vi "Process.vi"(8 "error in":errorcluster, 11 "Sequence Experiment UI":refnum<class "Control Experiment UI.lvclass">) -> (0 "error out":errorcluster, 3 "Sequence Experiment UI out":refnum<class "Control Experiment UI.lvclass">)   [LabVIEW 2019, in "Control Experiment UI.lvclass"]
doc: "---------------------------------------------------------------\nJKI State Machine Objects™\nhttp://jki.net/state-machine-objects/\nCopyright (C) 2005-2015, JKI <info@jki.net>\nALL RIGHTS RESERVEDJKI State Machine Objects (SMO) 1.0.0.5\nJKI - JKI\nCopyright (c) 2016, JKI"
uses:
  Control Experiment UI.lvclass
  <vilib>/JKI/JKI SMO/SMO/SMO.lvclass
  <vilib>/JKI/JKI SMO/SMO/Typedefs/Parent Call--Enum.ctl
  <vilib>/JKI/JKI SMO/SMO.UI/SMO.UI.lvclass
  <userlib>/LevyLab/Instrument Framework/SMOs/Instrument/Instrument.lvclass
  <userlib>/LevyLab/Instrument Framework/SMOs/Instrument UI/Instrument UI.lvclass
  Control Experiment/Control Experiment.lvclass
  <userlib>/LevyLab/Krohn Hite 7008/typedefs/Input Configuration-Enum.ctl
  <userlib>/LevyLab/Krohn Hite 7008/Instrument.KH7008.lvclass
  <userlib>/LevyLab/Instrument Framework/SMOs/Configuration/Configuration.lvclass
  Control Experiment/Private/Control Experiment SM/Typedefs/Instrument--enum.ctl
  Control Experiment/Private/Control Experiment SM/Typedefs/KH Mode-enum.ctl
  <userlib>/LevyLab/Krohn Hite 7008/typedefs/Gain-Enum.ctl
  <userlib>/LevyLab/Krohn Hite 7008/typedefs/Shunt-Enum.ctl
  Typedefs/UI Channels.AO--Cluster.ctl
  Typedefs/UI Channels.KH--Cluster.ctl
  Typedefs/UI Channels.Device--Cluster.ctl
  Typedefs/UI Channels.AI--Cluster.ctl
  Typedefs/UI Channels--Cluster.ctl
  Typedefs/UI Config--Cluster.ctl
  Control Experiment SM/Control Experiment SM.lvclass
  <userlib>/_OpenG.lib/array/array.llb/Remove Duplicates from 1D Array (Variant)__ogtk.vi
  C:/Program Files (x86)/National Instruments/LabVIEW 2016/user.lib/LevyLab/Levylab Instruments/SMOs/Instrument UI/Instrument UI.lvclass
  C:/Program Files (x86)/National Instruments/LabVIEW 2016/vi.lib/JKI/JKI SMO/SMO/SMO.lvclass
  C:/Program Files (x86)/National Instruments/LabVIEW 2016/vi.lib/JKI/JKI SMO/SMO.UI/SMO.UI.lvclass
  <userlib>/LevyLab/Krohn Hite 7008/typedefs/Filter-Enum.ctl
  <userlib>/LevyLab/Krohn Hite 7008/typedefs/Coupling-Enum.ctl
  C:/Program Files (x86)/National Instruments/LabVIEW 2016/user.lib/LevyLab/Levylab Instruments/SMOs/Instrument/Instrument.lvclass
panel:
  in  "Save Preset":bool
  in  "Load Preset":bool
  in  "KH Config Preset":string="A"
  in  "Number of AI":i32=8 caption="#AI"
  in  "Tab Control":enum32{"Input", "Configuration", "UI", "Output"}(tab)
  in  "UI Channels []":T1[](array[typedef]) {"KH"."Channel" items=["KH8 Ch8"]}
  in  "Default Gain":T7=enum."10x"
  in  "Krohn Hite?":bool=TRUE
  in  "Strain Cell?":bool=TRUE
  in  "C Bridge?":bool=TRUE
  in  "Lockin Address":string
  in  "Capacitance Bridge Address":refnum<visa-resource-name>
  in  "Strain Cell Address":refnum<visa-resource-name>
  in  "KH Addresses":refnum<visa-resource-name>[](array[refnum]) caption="KH Address[A,B,C,...]"
  in  "Default Shunt Resistor":T8=enum."50k Ohms"
  in  "KH All Buttons":T10(radio)
  in  "Bandwidth Filter":T11=enum."ON"
  in  "Coupling":T12=enum."DC"
  in  "Default Path":path=path "C:/DataTemp" caption="Base Path (Do not add your instrument name here)(Typ. G:\\My Drive\\ansom\\Data)"
  in  "Electrode Labels":string="n.c\nI1+\nI1-\nI2+\nI2-\nI3+\nI3-\nV1+\nV2-\nV2+\nV2-\nV3+\nV3-\ndV1\ndV2\ndV3\nVsg1\nVsg2\nVbg\n"
  out "Device Folder":path=path "G:/My Drive/ansom/Data/AGILENT/TEST.20200113" caption="(\\base path\\project\\device\\ )"
  out "Comments":string="Device: \r  Device Name: TEST.20200113\r  Computer: ASTARTES\r  User: Patrick\r  Instrument: AGILENT\r  Description: |\r    this is a test\r\rExperiment: \r  Time: 2020-02-25T09:02:18\r  Description: |\r\rSweep: \r- Loop1: [OFF, 0.000000]\r- Loop2: [OFF, 0.000000]\r- Loop3: [OFF, 0.000000]\r- Loop4: [OFF, 0.000000]\r\rWiring: \r- Electrode 27: Lockin 1, I+, KH1 Channel 1, Differential, 1x, 50k Ohms\r\rLockin: \r  AO: \r  \r  REF: \r  \r  Sampling: \r  - Fs: \r  - N: \r"
  in  "Create Output":bool
  in  "Description":string="this is a test"
  in  "Sample":string="TEST" caption="Sample (SAXXXX)"
  in  "Device Date":string="20200113" caption="Date (YYYYMMDD)"
  in  "Instrument":T13
  in  "Username":string="Patrick"
  in  "Experiment VIs":u16(ring) items=["----Sweep Control----", "Sweep Control.vi", "Continuous B Sweep.vi", "----Transport----", "IV.vi", "IV_Sweep.vi", "Lockin_time.vi", "Lockin_Vsg.vi", "Lockin_sweep.vi", "Lockin_AIWFM_time.vi", "THz_TimeDelay.vi", "Sweep_AIWFM_time.vi"]
  in  "Open VI":bool
  in  "Open Lockin":bool
  in  "STOP":bool
  in  "Blinking String":string
  # "Device and Project Description"
  # "Experiment VIs"
  # "Lockin (Local)"
  # "SMO UI Template"
  # "For instructions on how to use the JKI State Machine Objects, examples and video tutorials, visit:\nhttp://jki.net/state-machine-objects/\n\nJKI State Machine Objects™\nhttp://jki.net/state-machine-objects/\nCopyright (C) 2005-2015, JKI <info@jki.net>\nALL RIGHTS RESERVED"
  # "Output"
  # "Input"
  # "Device"
  # "Krohn Hite"
  # "Ch"
  # "Gain"
  # "Electrode"
  # "Label"
  # "Configuration"
  # "Ch"
  # "Configuration"
  # "Gain"
  # "Shunt Resistor"
  # "Ch"
  # "Gain"
  # "Krohn Hite Configuration"
  # "Hardware Configuration"
  # "Lockin"
  # "Path Configuration"
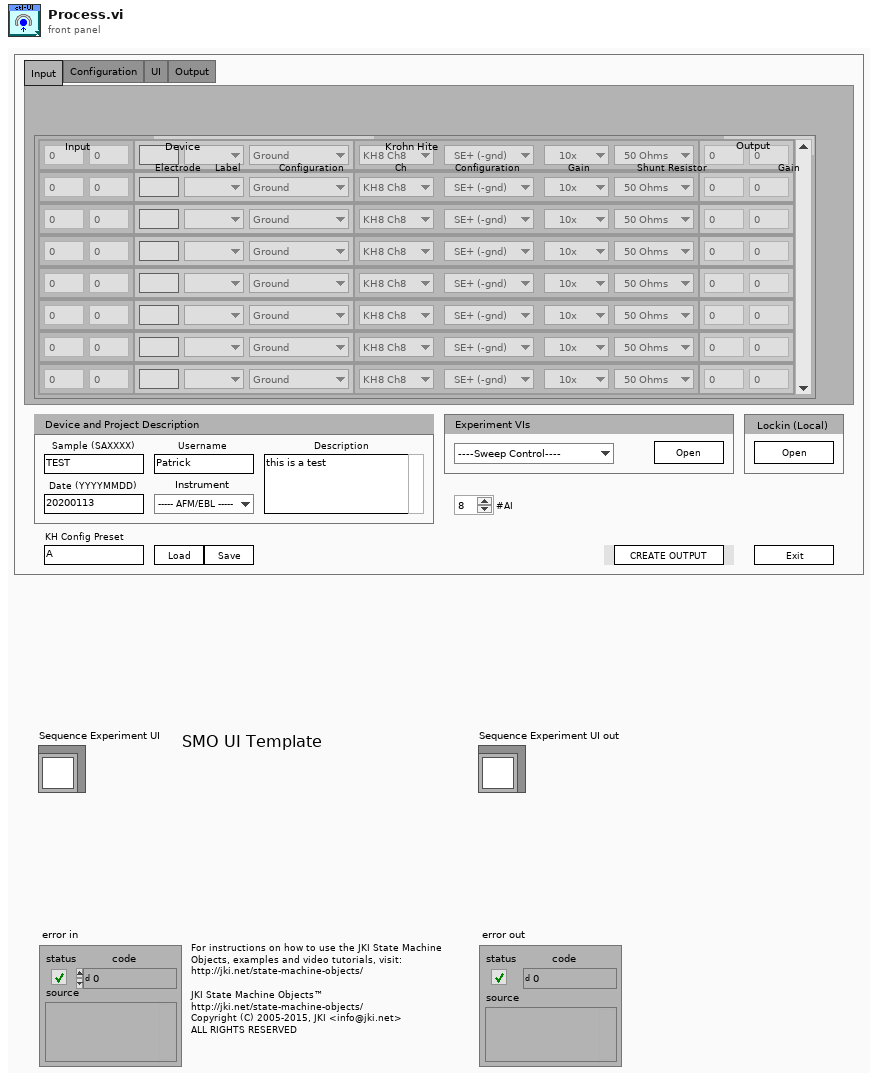
[diagram p1: front panel]
types:
  T1 = typedef "Control Experiment UI.lvclass/UI Channels--Cluster.ctl" = cluster{"AI":T2, "Device":T3, "KH":T5, "AO":T9}
  T2 = typedef "Control Experiment UI.lvclass/UI Channels.AI--Cluster.ctl" = cluster{"Channel":u32, "Gain":dbl}
  T3 = typedef "Control Experiment UI.lvclass/UI Channels.Device--Cluster.ctl" = cluster{"Electrode":string, "Configuration":T4, "Label":u16}
  T4 = typedef "Control Experiment.lvclass/KH Mode-enum.ctl" = enum16{"Ground", "Current", "Voltage (SE)", "Voltage (Diff)", "Gate"}
  T5 = typedef "Control Experiment UI.lvclass/UI Channels.KH--Cluster.ctl" = cluster{"Channel":u16, "Configuration":T6, "Gain":T7, "Shunt Resistor":T8}
  T6 = typedef "Instrument.KH7008.lvclass/Input Configuration-Enum.ctl" = enum16{"Ground", "SE+ (-gnd)", "SE- (+gnd)", "Differential"}
  T7 = typedef "Instrument.KH7008.lvclass/Gain-Enum.ctl" = enum16{"1x", "10x", "100x", "1000x"}
  T8 = typedef "Instrument.KH7008.lvclass/Shunt-Enum.ctl" = enum16{"Open", "50 Ohms", "500 Ohms", "5k Ohms", "50k Ohms", "10M Ohm"}
  T9 = typedef "Control Experiment UI.lvclass/UI Channels.AO--Cluster.ctl" = cluster{"Channel":u32, "Gain":dbl}
  T10 = enum32{"No Selection", "All Ground", "All Differential"}
  T11 = typedef "Instrument.KH7008.lvclass/Filter-Enum.ctl" = enum16{"OFF", "ON"}
  T12 = typedef "Instrument.KH7008.lvclass/Coupling-Enum.ctl" = enum16{"AC", "DC"}
  T13 = typedef "Control Experiment.lvclass/Instrument--enum.ctl" = enum16{"----- AFM/EBL -----", "AGILENT", "CYPHER", "Gemini2", "JEOL", "MFP3D", "----- Cryostat -----", "CF900", "DR200", "MNK", "PPMS 1", "PPMS 2", "PPMS 3", "----- Optics -----", "THz 1", "THz 2"}
  T14 = typedef "SMO.lvclass/Parent Call--Enum.ctl" = enum16{"Allows parent to run", "Does not request parent to run"}
  T15 = enum32{"invalid app kind", "Development System", "Run Time System", "Student Edition", "Embedded LabVIEW", "Evaluation", "Custom"}
  T16 = enum32{"Invalid", "Standard", "Closed", "Hidden", "Minimized", "Maximized"}
  T17 = typedef "Control Experiment.lvclass/UI Config--Cluster.ctl" = cluster{"Metadata":cluster{"Sample (SAXXXX)":string, "Device (YYYYMMDD)":string, "Description":string, "Username":string, "Default Path":path}, "Number of AI":i32, "UI Channels []":T1[], "Instruments":cluster{"Lockin Address":string, "Krohn Hite?":bool, "KH Addresses":refnum<visa-resource-name>[], "Strain Cell?":bool, "Strain Cell Address":refnum<visa-resource-name>, "C Bridge?":bool, "Capacitance Bridge Address":refnum<visa-resource-name>, "Instrument":T18}, "Krohn Hite":cluster{"Defualt Shunt Resistor":T8, "Default Gain":T7, "Coupling":T12, "Bandwidth Filter":T11}}
  T18 = typedef "Control Experiment SM.lvclass/Instrument--enum.ctl" = enum16{"----- AFM/EBL -----", "AGILENT", "CYPHER", "Gemini2", "JEOL", "MFP3D", "----- Cryostat -----", "CF900", "DR200", "MNK", "PPMS 1", "PPMS 2", "PPMS 3", "----- Optics -----", "THz 1", "THz 2"}
  T19 = cluster{"Core":cluster{"Current VI Reference":refnum<vi>, "Close Panel on Exit?":bool, "error":errorcluster}, "Instrument UI":refnum<class "Control Experiment UI.lvclass">, "Instrument":refnum<class "Control Experiment.lvclass">, "Number of AI":i32, "UI Channels []":T1[], "VI paths":path[], "Config":refnum<class "Configuration.lvclass">, "UIconfig":T17, "C.E.":refnum<class "Control Experiment SM.lvclass">, "SR":enum16{"500", "10M"}}
  T20 = typedef "Control Experiment.lvclass/PublicEvents--Control Experiment.getKHShuntType.ctl" = enum16{"500", "10M"}
  T21 = cluster{"Current VI Reference":refnum<vi>, "Close Panel on Exit?":bool, "error":errorcluster}
  T22 = typedef "SMO.lvclass/Protected Events.ctl" = cluster{"StopProcesses":refnum<user-event>, "AbortProcesses":refnum<user-event>, "Config Changed":refnum<user-event>, "Dependency":refnum<user-event>}
  T23 = typedef "Instrument.lvclass/PublicEvents--Cluster.ctl" = cluster{"MessageFromProcess":refnum<user-event>}
  T24 = typedef "Control Experiment.lvclass/PublicEvents--Cluster.ctl" = cluster{"getUIconfig":refnum<user-event>, "getKHShuntType":refnum<user-event>}
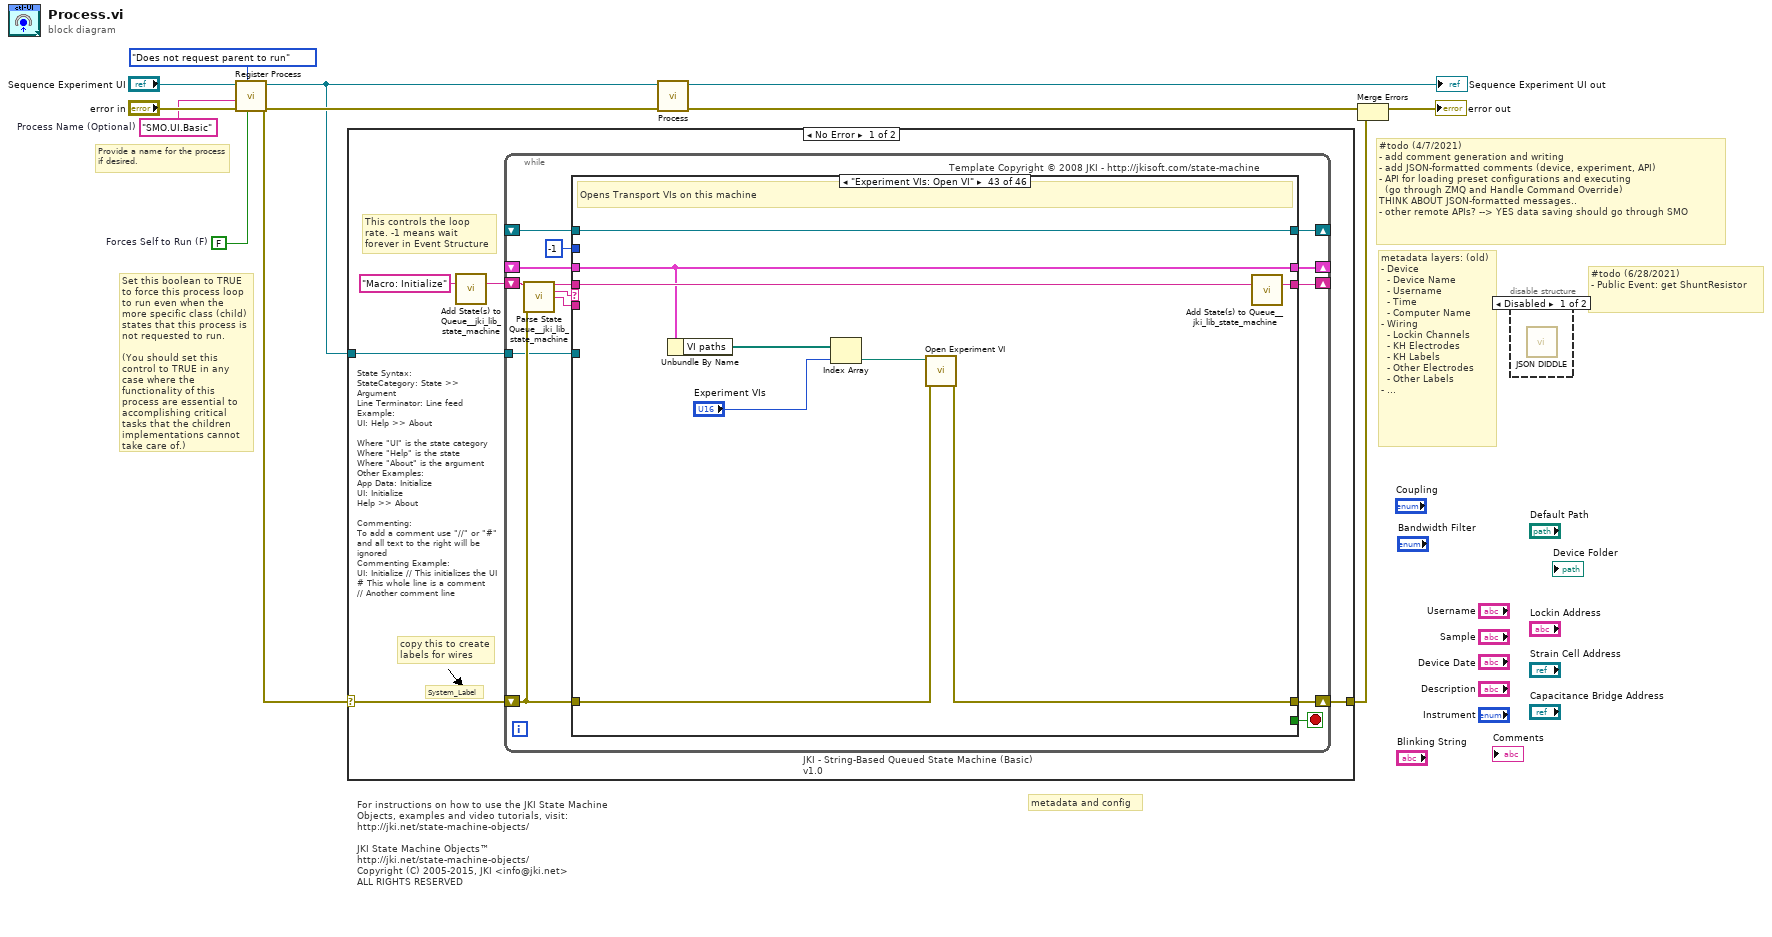
[diagram p0: block diagram]
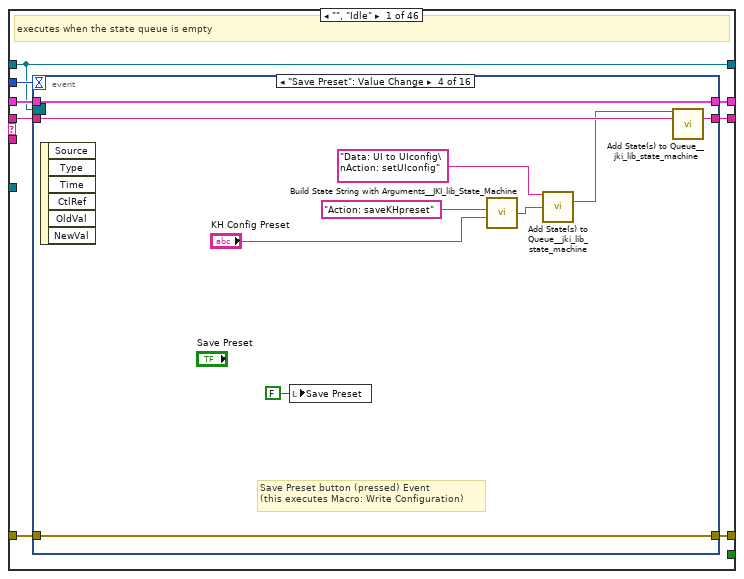
[diagram p3: hidden frame]
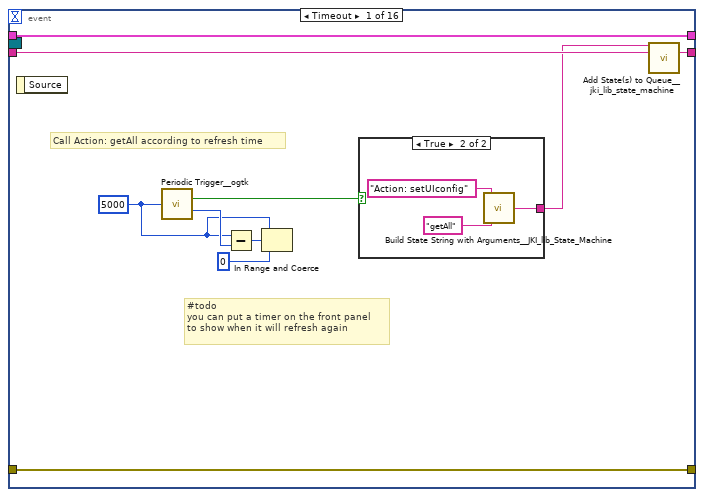
[diagram p4: hidden frame]
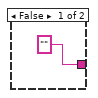
[diagram p5: hidden frame]
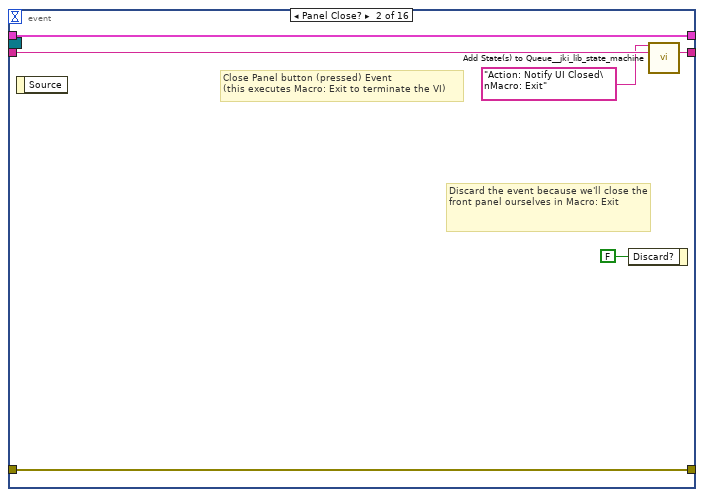
[diagram p6: hidden frame]
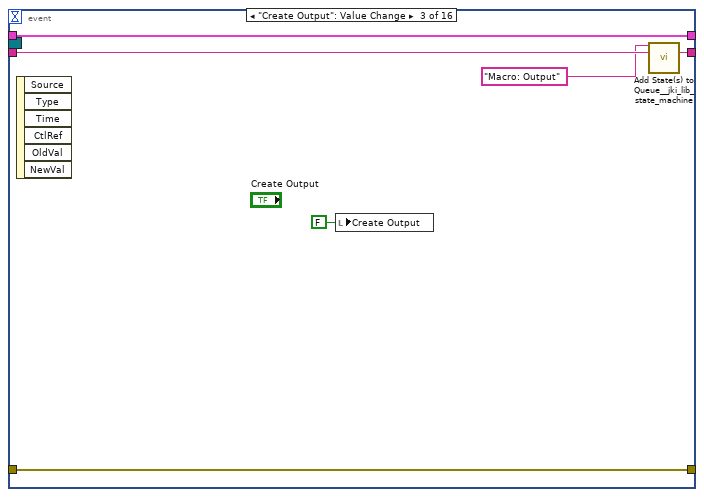
[diagram p7: hidden frame]
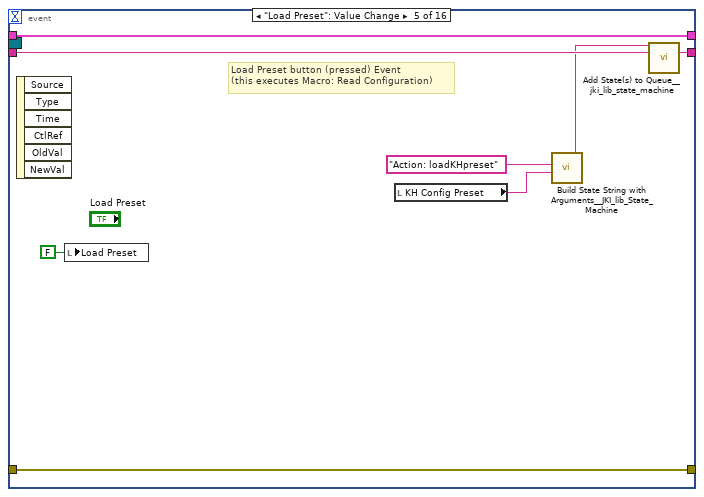
[diagram p8: hidden frame]
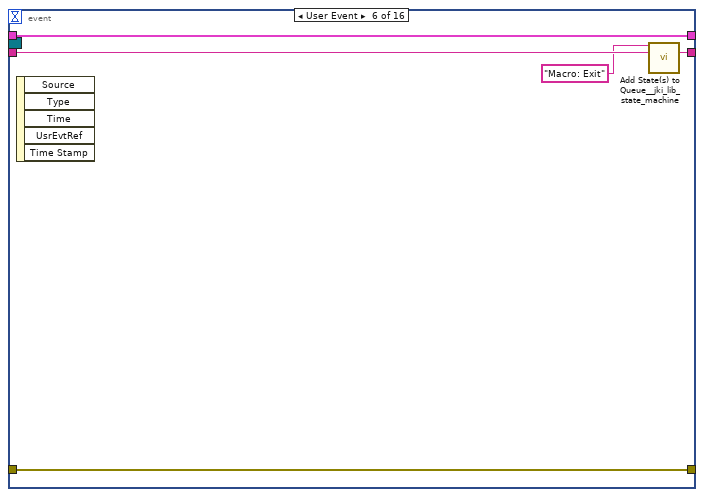
[diagram p9: hidden frame]
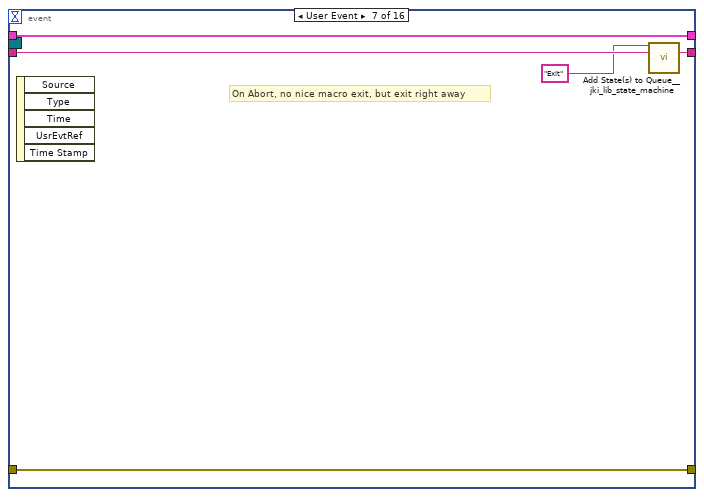
[diagram p10: hidden frame]
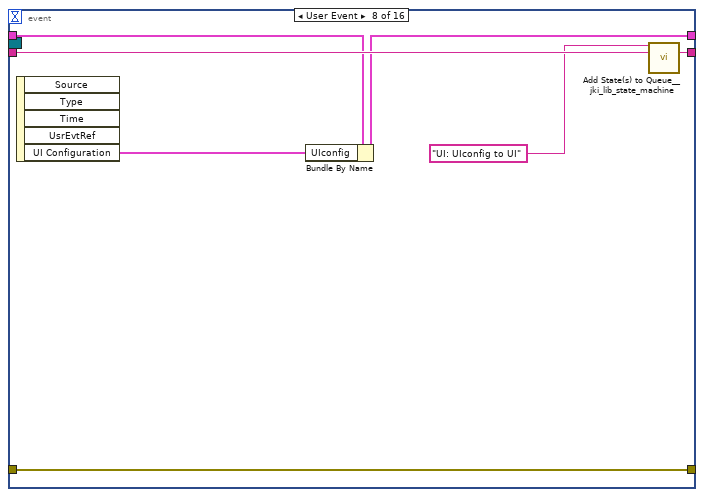
[diagram p11: hidden frame]
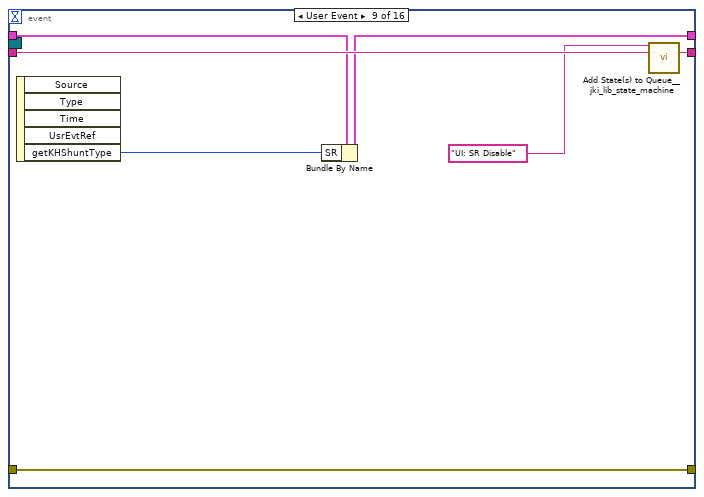
[diagram p12: hidden frame]
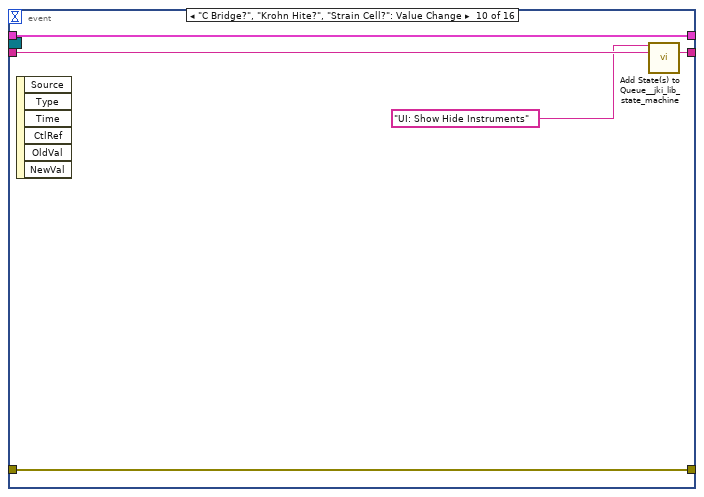
[diagram p13: hidden frame]
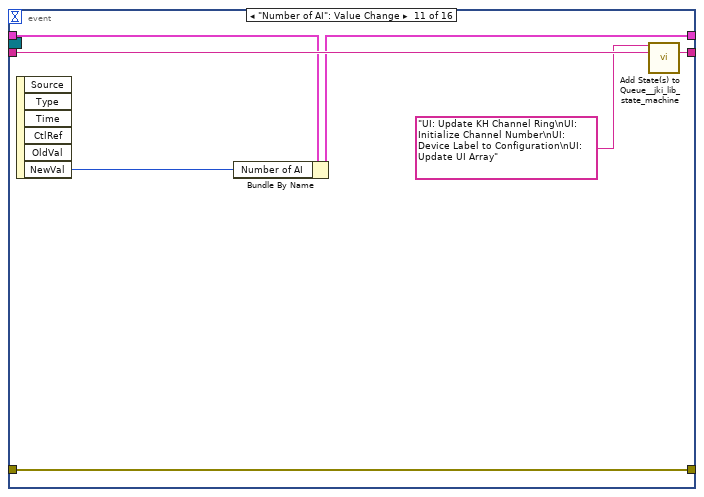
[diagram p14: hidden frame]
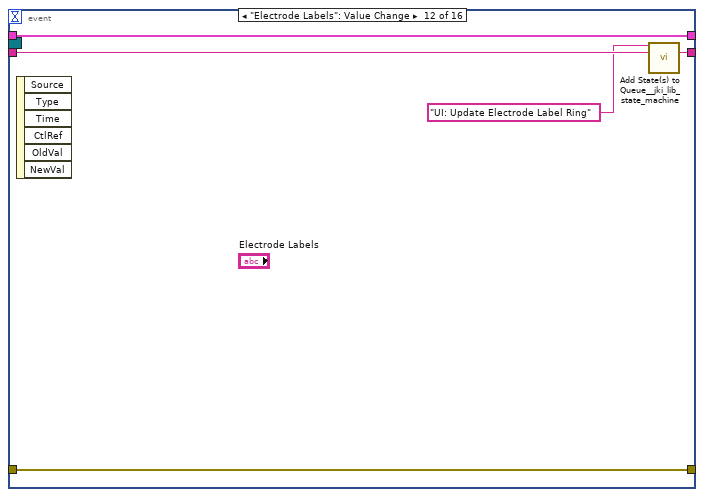
[diagram p15: hidden frame]
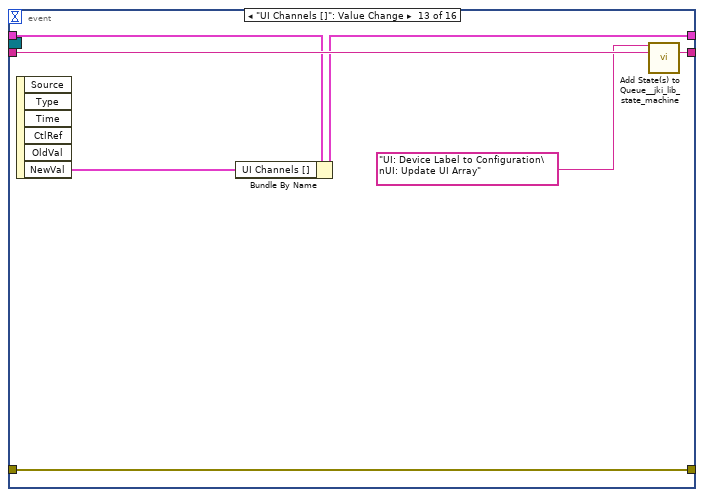
[diagram p16: hidden frame]
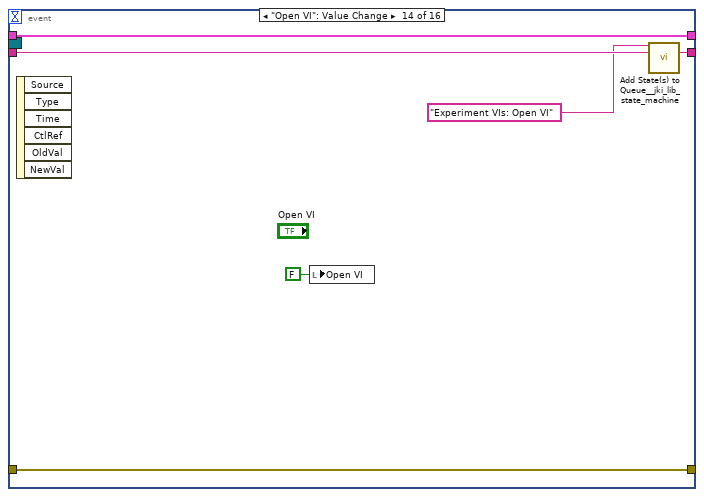
[diagram p17: hidden frame]
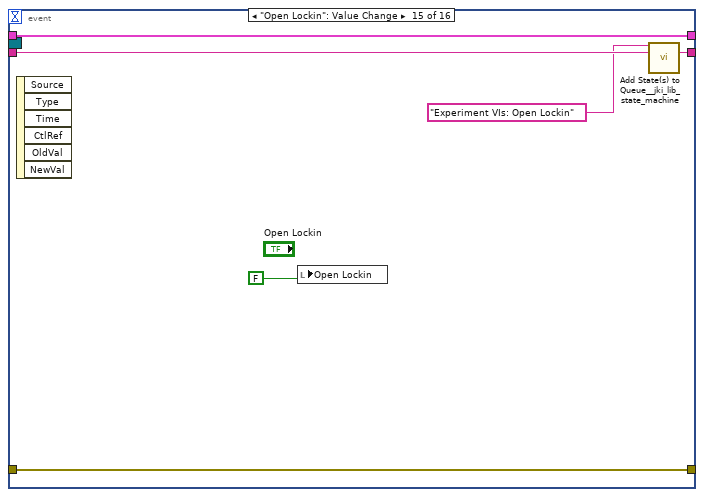
[diagram p18: hidden frame]
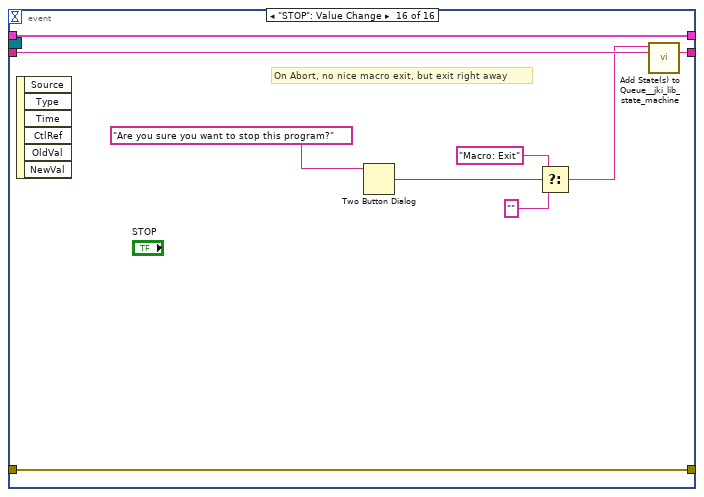
[diagram p19: hidden frame]
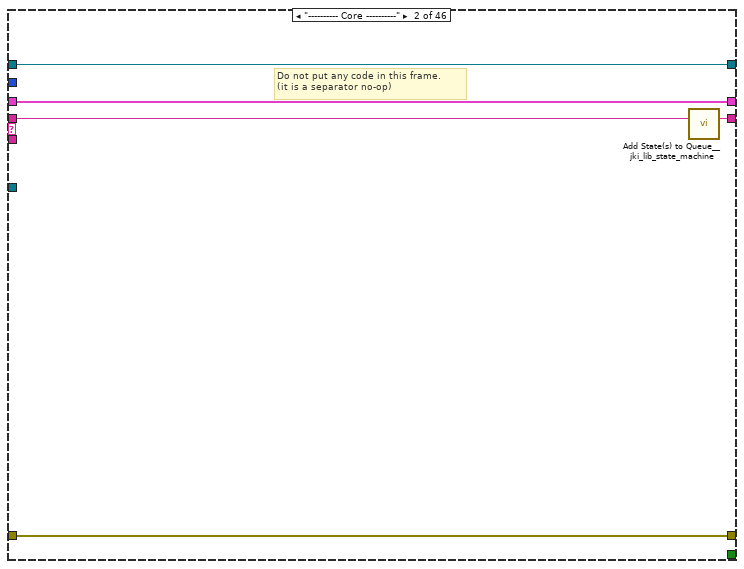
[diagram p20: hidden frame]
diagram:
  w2 = FALSE  # Forces Self to Run (F)
  w1 = "SMO.UI.Basic"  # Process Name (Optional)
  # "#todo (6/28/2021)\n- Public Event: get ShuntResistor"
  # "metadata layers: (old)\n- Device\n  - Device Name\n  - Username\n  - Time\n  - Computer Name\n- Wiring\n  - Lockin Channels\n  - KH Electrodes\n  - KH Labels\n  - Other Electrodes\n  - Other Labels\n- ..."
  # "#todo (4/7/2021)\n- add comment generation and writing\n- add JSON-formatted comments (device, experiment, API)\n- API for loading preset configurations and executing\n  (go through ZMQ and Handle Command Override)\nTHINK ABOUT JSON-formatted messages..\n- other remote APIs? --> YES data saving should go through SMO"
  # "metadata and config"
  # "Provide a name for the process\nif desired."
  # "Set this boolean to TRUE to force this process loop to run even when the more specific class (child) states that this process is not requested to run.\n\n(You should set this control to TRUE in any case where the functionality of this process are essential to accomplishing critical tasks that the children implementations cannot take care of.)"
  # "For instructions on how to use the JKI State Machine Objects, examples and video tutorials, visit:\nhttp://jki.net/state-machine-objects/\n\nJKI State Machine Objects™\nhttp://jki.net/state-machine-objects/\nCopyright (C) 2005-2015, JKI <info@jki.net>\nALL RIGHTS RESERVED"
  n1 = call <vilib>:"Register Process.vi"("Forces Self to Run (F)"=w2, "Parent Call"=Parent_Call--Enum."Does not request parent to run", "error in (no error)"="error in", "Process Name (optional)"=w1, "SMO"="Sequence Experiment UI") -> ("error out"=w8:errorcluster, "SMO out"=w7:refnum<class "Control Experiment UI.lvclass">)  [unwired: 5 in]
  n2 = case shown="No Error" w8 {
    selector: w8 -> [w13 w653]
    tunnel: w7 -> [w14 _]
    tunnel: [w12 w653] -> w4
    frame No Error {
      # "State Syntax:\nStateCategory: State >> Argument\nLine Terminator: Line feed\nExample:\nUI: Help >> About\n\nWhere \"UI\" is the state category\nWhere \"Help\" is the state\nWhere \"About\" is the argument\nOther Examples:\nApp Data: Initialize\nUI: Initialize\nHelp >> About\n\nCommenting:\nTo add a comment use \"//\" or \"#\" and all text to the right will be ignored\nCommenting Example:\nUI: Initialize // This initializes the UI\n# This whole line is a comment\n// Another comment line"
      # "copy this to create labels for wires"
      # "This controls the loop rate. -1 means wait forever in Event Structure"
      # "System_Label"
      n3 = call <vilib>:"Add State(s) to Queue__jki_lib_state_machine.vi"("State(s) in (\"\")"="Macro: Initialize") -> ("States Out"=w16:string)  [unwired: 14 in]
      n4 = while "JKI - String-Based Queued State Machine (Basic) v1.0" {
        shift-right: [w23] -> _
        shift-left: _ -> [w22]
        shift-right: [w26] -> w12
        shift-left: w13 -> [w20]
        shift-right: [w25] -> _
        shift-left: w16 -> [w27]
        tunnel: w14 -> [w19]
        shift-right: [w18] -> _
        shift-left: _ -> [w17]
        stop <- w24 stop-if-true
        # "Template Copyright © 2008 JKI - http://jkisoft.com/state-machine"
        n5 = call <vilib>:"Parse State Queue__jki_lib_state_machine.vi"("State Queue"=w27, "Error In (no error)"=w20) -> ("Remaining States"=w29:string, "Current State"=w30:string, "Arguments"=w28:string)  [unwired: 11 in]
        n6 = case shown="\"Experiment VIs: Open VI\"" w30 {
          selector: w30 -> [_ _ w158 _ _ _ _ _ _ _ _ _ _ _ _ _ _ _ _ _ _ _ _ _ _ _ _ _ _ _ _ _ _ _ _ _ _ _ _ _ _ _ _ _ _ _]
          tunnel: w29 -> [w38 w156 w162 w181 w195 w201 w206 w228 w253 w260 w265 w274 w283 w293 w304 w325 w339 w349 w358 w371 w397 w403 w410 w426 w458 w467 w473 w479 w494 w499 w510 w517 w522 w538 w544 w551 w558 w566 w574 w582 w589 w612 w627 w633 w640 w651]
          tunnel: w28 -> [_ _ _ _ _ _ _ _ _ _ _ _ _ _ _ _ _ _ w350 _ _ _ w404 w420 _ _ _ _ _ _ _ _ _ _ _ _ _ _ w567 w575 _ _ _ _ _ _]
          tunnel: w22 -> [w36 w153 w160 w172 w184 w197 w203 _ w230 w255 w262 w272 w281 w285 w299 w322 w336 w341 w355 w368 w393 w399 w408 w422 w455 w463 w470 w476 w481 w496 w507 w512 w519 w536 w542 w547 w554 w563 w571 w579 w585 w608 w619 w630 w636 w644]
          tunnel: [w35 w154 w164 w178 w186 w196 w204 w218 w251 w256 w263 w269 w275 w287 w302 w314 w331 w345 w356 w369 w395 w401 w405 w423 w456 w465 w471 w477 w492 w497 w501 w513 w520 w531 w539 w548 w552 w559 w568 w576 w586 w609 w620 w628 w637 w641] -> w26
          tunnel: w20 -> [w34 w154 w163 w178 w191 _ w204 w225 w251 w257 w263 w270 w276 w289 w302 w315 w333 w342 w356 w369 w395 w401 w406 w424 w456 w465 w471 w477 w492 w497 w502 w514 w520 w533 w540 w548 w553 w560 w569 w577 w586 w609 w621 w629 w637 w646]
          tunnel: [w37 w155 w161 w180 w194 w200 w205 w227 w252 w259 w264 w273 w282 w292 w303 w324 w338 w348 w357 w370 w396 w402 w409 w425 w457 w466 w472 w478 w493 w498 w509 w516 w521 w537 w543 w550 w557 w565 w573 w581 w588 w611 w626 w632 w639 w650] -> w25
          tunnel: [_ _ _ _ _ TRUE _ _ _ _ _ _ _ _ _ _ _ _ _ _ _ _ _ _ _ _ _ _ _ _ _ _ _ _ _ _ _ _ _ _ _ _ _ _ _ _] -> w24
          tunnel: [w33 w153 w160 w179 w183 w197 w203 w226 w229 w255 w262 w272 w281 w285 w298 w321 w336 w341 w355 w368 w393 w399 w408 w422 w455 w463 w470 w476 w481 w496 w507 w512 w519 w536 w542 w546 w554 w563 w571 w579 w583 w607 w619 w630 w634 w643] -> w23
          tunnel: -1 ("Timeout") -> [w32 _ _ _ _ _ _ _ _ _ _ _ _ _ _ _ _ _ _ _ _ _ _ _ _ _ _ _ _ _ _ _ _ _ _ _ _ _ _ _ _ _ _ _ _ _]
          tunnel: w19 -> [_ _ _ _ _ _ _ w223 _ _ _ _ _ _ _ _ _ _ _ _ _ _ _ _ _ _ _ _ _ _ _ _ _ _ _ _ _ _ _ _ _ _ _ _ _ _]
          tunnel: [w31 w152 w157 w169 w193 w198 w202 w222 w250 w254 w261 w271 w280 w291 w301 w323 w337 w347 w354 w367 w394 w400 w407 w419 w454 w464 w469 w475 w486 w495 w508 w515 w518 w535 w541 w549 w556 w564 w572 w580 w587 w610 w625 w631 w638 w649] -> w18
          tunnel: w17 -> [w31 w152 w157 w169 w193 w198 w202 w222 w250 w254 w261 w271 w280 w291 w301 w323 w337 w347 w354 w367 w394 w400 w407 w419 w454 w464 w469 w475 w486 w495 w508 w515 w518 _ w541 w549 w556 w564 w572 w580 w587 w610 w625 w631 w638 w649]
          frame "", "Idle" {
            # "executes when the state queue is empty"
            n7 = event shown="[3] \"Save Preset\": Value Change" {
              selector: w31 -> [_ _ _ _ _ _ _ _ _ _ _ _ _ _ _ _]
              dyn-events: _ -> [_ _ _ _ _ _ _ _ _ _ _ _ _ _ _ _]
              timeout: w32 -> [_ _ _ _ _ _ _ _ _ _ _ _ _ _ _ _]
              tunnel: w38 -> [w48 w58 w64 w74 w82 w87 w92 w99 w106 w111 w118 w123 w130 w136 w142 w151]
              tunnel: [w47 w57 w63 w73 w81 w86 w91 w98 w105 w110 w117 w122 w129 w135 w141 w150] -> w37
              tunnel: w36 -> [w45 w54 w61 w71 w79 w84 w89 w95 w102 w108 w113 w120 w126 w133 w139 w148]
              tunnel: [w46 w53 w60 w70 w76 w85 w90 w97 w104 w109 w116 w121 w128 w134 w140 w149] -> w35
              tunnel: w34 -> [w46 w53 w60 w70 w76 w85 w90 w97 w104 w109 w116 w121 w128 w134 w140 w149]
              tunnel: [w45 w54 w61 w71 w79 w84 w89 w94 w101 w108 w112 w120 w125 w133 w139 w148] -> w33
              event Timeout {
                w40 = u32 5000 ("time (ms)")
                # "#todo\nyou can put a timer on the front panel\nto show when it will refresh again"
                # "Call Action: getAll according to refresh time"
                n8 = event-data() -> ()  [unwired: 1 in, 1 out]
                n9 = call <userlib>:"Periodic Trigger__ogtk.vi"("time (ms)"=w40) -> ("Triggered"=w43:bool, "timer value"=w42:u32)  [unwired: 12 in, 1 out]
                n10 = Subtract(x=w40, y=w42) -> (x-y=w41:u32)
                n11 = In Range and Coerce(upper limit=w40, x=w41, lower limit=u32 0) -> ()  [unwired: 2 out]
                n12 = case shown="True" w43 {
                  tunnel: ["" ("State(s) in Front (\"\")") w50] -> w44
                  frame False {
                  }
                  frame True {
                    n13 = call <vilib>:"Build State String with Arguments__JKI_lib_State_Machine.vi"("Arguments (\"\")"="getAll" ("State(s) in Front (\"\")"), "State"="Action: setUIconfig" ("State(s) in Front (\"\")")) -> ("State with Arguments"=w50:string)  [unwired: 4 in]
                  }
                }
                n14 = call <vilib>:"Add State(s) to Queue__jki_lib_state_machine.vi"("State(s) in Front (\"\")"=w44, "State(s) in (\"\")"=w48) -> ("States Out"=w47:string)  [unwired: 13 in]
              }
              event Panel Close? {
                # "Discard the event because we'll close the front panel ourselves in Macro: Exit"
                # "Close Panel button (pressed) Event\n(this executes Macro: Exit to terminate the VI)"
                n15 = event-data() -> ()  [unwired: 1 in, 1 out]
                n16 = event-data("Discard?"=FALSE) -> ()  [unwired: 1 in, 1 out]
                n17 = call <vilib>:"Add State(s) to Queue__jki_lib_state_machine.vi"("State(s) in Front (\"\")"="Action: Notify UI Closed\nMacro: Exit", "State(s) in (\"\")"=w58) -> ("States Out"=w57:string)  [unwired: 13 in]
              }
              event "Create Output": Value Change {
                n18 = event-data() -> ()  [unwired: 1 in, 6 out]
                n19 = local write "Create Output"(FALSE ("Create Output")) -> ()
                n20 = call <vilib>:"Add State(s) to Queue__jki_lib_state_machine.vi"("State(s) in Front (\"\")"="Macro: Output", "State(s) in (\"\")"=w64) -> ("States Out"=w63:string)  [unwired: 13 in]
              }
              event "Save Preset": Value Change {
                # "Save Preset button (pressed) Event\n(this executes Macro: Write Configuration)"
                n21 = event-data() -> ()  [unwired: 1 in, 6 out]
                n22 = local write "Save Preset"(FALSE ("Save Preset")) -> ()
                n23 = call <vilib>:"Build State String with Arguments__JKI_lib_State_Machine.vi"("Arguments (\"\")"="KH Config Preset", "State"="Action: saveKHpreset") -> ("State with Arguments"=w67:string)  [unwired: 4 in]
                n24 = call <vilib>:"Add State(s) to Queue__jki_lib_state_machine.vi"("State(s) in Front (\"\")"="Data: UI to UIconfig\nAction: setUIconfig" ("State(s) in Front (\"\")"), "State(s) at Back (\"\")"=w67) -> ("States Out"=w66:string)  [unwired: 13 in]
                n25 = call <vilib>:"Add State(s) to Queue__jki_lib_state_machine.vi"("State(s) in Front (\"\")"=w66, "State(s) in (\"\")"=w74) -> ("States Out"=w73:string)  [unwired: 13 in]
              }
              event "Load Preset": Value Change {
                # "Load Preset button (pressed) Event\n(this executes Macro: Read Configuration)"
                n26 = event-data() -> ()  [unwired: 1 in, 6 out]
                n27 = local write "Load Preset"(FALSE ("Load Preset")) -> ()
                n28 = local read "KH Config Preset"() -> (w75:string)
                n29 = call <vilib>:"Build State String with Arguments__JKI_lib_State_Machine.vi"("Arguments (\"\")"=w75, "State"="Action: loadKHpreset") -> ("State with Arguments"=w77:string)  [unwired: 4 in]
                n30 = call <vilib>:"Add State(s) to Queue__jki_lib_state_machine.vi"("State(s) in Front (\"\")"=w77, "State(s) in (\"\")"=w82) -> ("States Out"=w81:string)  [unwired: 13 in]
              }
              event User Event {
                n31 = event-data() -> ()  [unwired: 1 in, 5 out]
                n32 = call <vilib>:"Add State(s) to Queue__jki_lib_state_machine.vi"("State(s) in Front (\"\")"="Macro: Exit", "State(s) in (\"\")"=w87) -> ("States Out"=w86:string)  [unwired: 13 in]
              }
              event User Event {
                # "On Abort, no nice macro exit, but exit right away"
                n33 = event-data() -> ()  [unwired: 1 in, 5 out]
                n34 = call <vilib>:"Add State(s) to Queue__jki_lib_state_machine.vi"("State(s) in Front (\"\")"="Exit", "State(s) in (\"\")"=w92) -> ("States Out"=w91:string)  [unwired: 13 in]
              }
              event User Event {
                n35 = event-data() -> ("UI Configuration"=w96:T17)  [unwired: 1 in, 4 out]
                n36 = Bundle By Name(cluster=w95, "UIconfig"=w96) -> (w94:T19)
                n37 = call <vilib>:"Add State(s) to Queue__jki_lib_state_machine.vi"("State(s) in Front (\"\")"="UI: UIconfig to UI" ("State(s) in Front (\"\")"), "State(s) in (\"\")"=w99) -> ("States Out"=w98:string)  [unwired: 13 in]
              }
              event User Event {
                n38 = event-data() -> ("getKHShuntType"=w103:T20)  [unwired: 1 in, 4 out]
                n39 = Bundle By Name(cluster=w102, "SR"=w103) -> (w101:T19)
                n40 = call <vilib>:"Add State(s) to Queue__jki_lib_state_machine.vi"("State(s) in Front (\"\")"="UI: SR Disable" ("State(s) in Front (\"\")"), "State(s) in (\"\")"=w106) -> ("States Out"=w105:string)  [unwired: 13 in]
              }
              event "C Bridge?", "Krohn Hite?", "Strain Cell?": Value Change {
                n41 = event-data() -> ()  [unwired: 1 in, 6 out]
                n42 = call <vilib>:"Add State(s) to Queue__jki_lib_state_machine.vi"("State(s) in Front (\"\")"="UI: Show Hide Instruments", "State(s) in (\"\")"=w111) -> ("States Out"=w110:string)  [unwired: 13 in]
              }
              event "Number of AI": Value Change {
                n43 = event-data() -> ("NewVal"=w114:i32)  [unwired: 1 in, 5 out]
                n44 = Bundle By Name(cluster=w113, "Number of AI"=w114) -> (w112:T19)
                n45 = call <vilib>:"Add State(s) to Queue__jki_lib_state_machine.vi"("State(s) in Front (\"\")"="UI: Update KH Channel Ring\nUI: Initialize Channel Number\nUI: Device Label to Configuration\nUI: Update UI Array", "State(s) in (\"\")"=w118) -> ("States Out"=w117:string)  [unwired: 13 in]
              }
              event "Electrode Labels": Value Change {
                n46 = event-data() -> ()  [unwired: 1 in, 6 out]
                n47 = call <vilib>:"Add State(s) to Queue__jki_lib_state_machine.vi"("State(s) in Front (\"\")"="UI: Update Electrode Label Ring", "State(s) in (\"\")"=w123) -> ("States Out"=w122:string)  [unwired: 13 in]
              }
              event "UI Channels []": Value Change {
                n48 = event-data() -> ("NewVal"=w124:T1[])  [unwired: 1 in, 5 out]
                n49 = Bundle By Name(cluster=w126, "UI Channels []"=w124) -> (w125:T19)
                n50 = call <vilib>:"Add State(s) to Queue__jki_lib_state_machine.vi"("State(s) in Front (\"\")"="UI: Device Label to Configuration\nUI: Update UI Array", "State(s) in (\"\")"=w130) -> ("States Out"=w129:string)  [unwired: 13 in]
              }
              event "Open VI": Value Change {
                n51 = event-data() -> ()  [unwired: 1 in, 6 out]
                n52 = local write "Open VI"(FALSE ("Open VI")) -> ()
                n53 = call <vilib>:"Add State(s) to Queue__jki_lib_state_machine.vi"("State(s) in Front (\"\")"="Experiment VIs: Open VI", "State(s) in (\"\")"=w136) -> ("States Out"=w135:string)  [unwired: 13 in]
              }
              event "Open Lockin": Value Change {
                n54 = event-data() -> ()  [unwired: 1 in, 6 out]
                n55 = local write "Open Lockin"(FALSE ("Open VI")) -> ()
                n56 = call <vilib>:"Add State(s) to Queue__jki_lib_state_machine.vi"("State(s) in Front (\"\")"="Experiment VIs: Open Lockin", "State(s) in (\"\")"=w142) -> ("States Out"=w141:string)  [unwired: 13 in]
              }
              event "STOP": Value Change {
                # "On Abort, no nice macro exit, but exit right away"
                n57 = event-data() -> ()  [unwired: 1 in, 6 out]
                n58 = Two Button Dialog(message="Are you sure you want to stop this program?") -> (T button?=w147:bool)  [unwired: 2 in]
                n59 = Select(t="Macro: Exit", s=w147, f="") -> (s? t:f=w143:string)
                n60 = call <vilib>:"Add State(s) to Queue__jki_lib_state_machine.vi"("State(s) in Front (\"\")"=w143, "State(s) in (\"\")"=w151) -> ("States Out"=w150:string)  [unwired: 13 in]
              }
            }
          }
          frame "---------- Core ----------" {
            # "Do not put any code in this frame.\n(it is a separator no-op)"
            n61 = call <vilib>:"Add State(s) to Queue__jki_lib_state_machine.vi"("State(s) in (\"\")"=w156) -> ("States Out"=w155:string)  [unwired: 14 in]
          }
          frame Default {
            w167 = 42 items=["No error", "Argument error", "Memory is full", "Out of zone", "End of file", "File already open", "Generic file I/O error", "File not found", "File permission error", "Disk is full", "Duplicate path", "Too many files open", "System feature not enabled", "Resource file not found", "Cannot add resource", "Resource not found", "Image not found", "Image memory error", "Pen does not exist", "Config type invalid", "Config token not found", "Config parse error", "Config memory error", "Bad external code format", "Bad external code offset", "External code not present", "Null window", "Destroy window error", "Null menu", "Print aborted", "Bad print record", "Print driver error", "Windows error during printing", "Memory error during printing", "Print dialog error", "Generic print error", "Invalid device refnum", "Device not found", "Device parameter error", "Device unit error", "Cannot open device", "Device call aborted", "Generic error", "Cancelled by user", "Object ID too low", "Object ID too high", "Object not in heap", "Unknown heap", "Unknown object (invalid DefProc)", "Unknown object (DefProc not in table)", "Message out of range", "Invalid (null) method", "Unknown message", "Manager call not supported", "Bad address", "Network operation in progress", "Network operation timed out", "Connection is busy", "Network attribute not supported", "Network error", "Address in use", "System out of memory", "Connection aborted", "Connection refused", "Not connected", "Already connected", "Connection closed", "Initialization error (interapplication manager)", "Bad occurrence", "Wait on unbound occurrence handler", "Occurrence queue overflow", "Datalog type conflict", "Unused", "Unrecognized type (interapplication manager)", "Memory corrupt", "Failed to make temporary DLL", "Old CIN version", "Drag socket not found", "Failed to load drop-object", "Failed to register OLE object", "Failed to release OLE object", "Format specifier type mismatch", "Unknown format specifier", "Too few format specifiers", "Too many format specifiers", "Scan failed", "Newer CIN version", "Error converting to variant", "Runtime menu error", "Password tampered", "Variant attribute not found", "Incompatible variant data type", "Event data is not available", "Event Store is not present", "Occurrence is not found", "Event Queue is not created", "Event info is not available", "Refnum passed is NULL", "Error retrieving Class GUID", "Error retrieving CoClass GUID", "Error retrieving TypeLib GUID.", "Bad built application magic bytes.", "Specific driver is different from the specific driver associated with the Logical Name.", "There is no session opened to the class driver.", "Max Error", "MAX - Error with config objects", "MAX - Error loading configuration", "MAX - Group not supported"]
            # "Current State"
            # "Do not delete, rename, or modify this frame.\n(this is used to capture unhandled states and typos)"
            # "Handle mistyped state name (developer tool)"
            n62 = Format Into String(format string="Software Exception: Unhandled State \"%s\"." ("message"), error in=w163, w158) -> (resulting string=w166:string, error out=w165:errorcluster)  [unwired: 1 in]
            n63 = call <vilib>:"Error Cluster From Error Code.vi"("show call chain? (False)"=TRUE, "error in (no error)"=w165, "error message (\"\")"=w166, "error code (0)"=w167) -> ("error out"=w164:errorcluster)  [unwired: 5 in]
            n64 = call <vilib>:"Add State(s) to Queue__jki_lib_state_machine.vi"("State(s) in (\"\")"=w162) -> ("States Out"=w161:string)  [unwired: 14 in]
          }
          frame "Initialize Core Data" {
            # "Do not delete, rename, or modify this frame.\n(this is used to determine panel behavior on exit)"
            # "originally closed?"
            # "exe?"
            # "If panel starts closed or is an EXE, then close it when we exit"
            n65 = property class="VI"() -> ("Front Panel.Open"=w177:bool)  [unwired: 2 in, 2 out]
            n66 = property class="App"() -> ("App.Kind"=w176:T15)  [unwired: 2 in, 2 out]
            n67 = control-ref of="Current VI Reference"() -> (w170:refnum<vi>)
            n68 = Not(x=w177) -> (.not. x?=w174:bool)
            n69 = Equal?(x=w176, y=T15."Run Time System" ("Application:Kind")) -> (x = y?=w173:bool)
            n70 = Or(x=w174, y=w173) -> (x .or. y?=w171:bool)
            n71 = Bundle By Name(cluster=w172, "Core.Current VI Reference"=w170, "Core.Close Panel on Exit?"=w171) -> (w179:T19)
            n72 = call <vilib>:"Add State(s) to Queue__jki_lib_state_machine.vi"("State(s) in (\"\")"=w181) -> ("States Out"=w180:string)  [unwired: 14 in]
          }
          frame "Error Handler" {
            w186 = errorcluster {"status"=FALSE, "code"=0, "source"=""}  # No error
            # "Overwrite this method to handle errors and pass to parent if not handled. Parent will fire a public event if the error is not handled up the chain of classes."
            # "Handle any errors here.\nYou can also output any states to clean-up after errors occur"
            n73 = Unbundle By Name(w184) -> ("Instrument UI"=w192:refnum<class "Control Experiment UI.lvclass">)
            n74 = call-dynamic "Handle Error.vi"("Stop on Unhandled Error (T)"=FALSE, "error in"=w191, "SMO"=w192) -> ("handling error"=w187:errorcluster, "Unhandled error"=w185:errorcluster)  [unwired: 6 in, 1 out]
            n75 = Bundle By Name(cluster=w184, "Core.error"=w185) -> (w183:T19)
            n76 = Select(t="Exit", s=w187, f="") -> (s? t:f=w188:string)
            n77 = call <vilib>:"Add State(s) to Queue__jki_lib_state_machine.vi"("State(s) in Front (\"\")"=w188, "State(s) in (\"\")"=w195) -> ("States Out"=w194:string)  [unwired: 13 in]
          }
          frame "Exit" {
            # "Do not put any code in this frame.\n(No errors that occur here will be handled.)"
            n78 = Unbundle By Name(w197) -> ("Core.error"=w196:errorcluster)
            n79 = call <vilib>:"Add State(s) to Queue__jki_lib_state_machine.vi"("State(s) in (\"\")"=w201) -> ("States Out"=w200:string)  [unwired: 14 in]
          }
          frame "---------- Data ----------" {
            # "Do not put any code in this frame.\n(It is a separator no-op. You can make a copy of this frame to create a new Data frame)"
            n80 = call <vilib>:"Add State(s) to Queue__jki_lib_state_machine.vi"("State(s) in (\"\")"=w206) -> ("States Out"=w205:string)  [unwired: 14 in]
          }
          frame "Data: Initialize" {
            w207 = enum16{"500", "10M"}."500"  # SR
            w212 = refnum<class "Control Experiment SM.lvclass"> refnum  # C.E.
            w214 = T17 {"Metadata"={"Sample (SAXXXX)"="", "Device (YYYYMMDD)"="", "Description"="", "Username"="", "Default Path"=path ""}, "Number of AI"=8, "UI Channels []"=[], "Instruments"={"Lockin Address"="", "Krohn Hite?"=TRUE, "KH Addresses"=[], "Strain Cell?"=TRUE, "Strain Cell Address"="", "C Bridge?"=TRUE, "Capacitance Bridge Address"="", "Instrument"=enum."----- AFM/EBL -----"}, "Krohn Hite"={"Defualt Shunt Resistor"=enum."50k Ohms", "Default Gain"=enum."10x", "Coupling"=enum."DC", "Bandwidth Filter"=enum."ON"}}  # UIconfig
            w213 = refnum<class "Configuration.lvclass"> refnum  # Config
            w215 = path[] []  # VI paths
            w216 = refnum<class "Control Experiment.lvclass"> refnum  # Instrument
            w221 = T21 {"Current VI Reference"=refnum, "Close Panel on Exit?"=FALSE, "error"={"status"=FALSE, "code"=0, "source"=""}}  # Core
            w224 = refnum<class "Control Experiment UI.lvclass"> refnum  # Self Reference
            # "typedef from Child Instrument"
            # "do not delete - used by framework"
            # "Data names and types of shift register data are defined by this bundle."
            # "Initialize the shift-register data, here.\n(data names are defined by what you wire into the bundle function)"
            n81 = Variant To Data(error in=w225, type=w224, Variant=w223) -> (data=w211:refnum<class "Control Experiment UI.lvclass">, error out=w219:errorcluster)
            n82 = call <userlib>:"Read Instrument.vi"("error in (no error)"=w219, "Instrument UI in"=w211) -> ("error out"=w218:errorcluster, "Instrument"=w217:refnum<class "Instrument.lvclass">, "Instrument UI"=w210:refnum<class "Control Experiment UI.lvclass">)  [unwired: 7 in]
            n83 = To More Specific Class(target class=w216, reference=w217) -> (specific class reference=w220:refnum<class "Control Experiment.lvclass">)  [unwired: 1 in, 1 out]
            n84 = Bundle("Core"=w221, "Instrument UI"=w210, "Instrument"=w220, "Number of AI"="Number of AI", "UI Channels []"="UI Channels []", "VI paths"=w215, "Config"=w213, "UIconfig"=w214, "C.E."=w212, "SR"=w207) -> (w226:T19)  [unwired: 1 in]
            n85 = call <vilib>:"Add State(s) to Queue__jki_lib_state_machine.vi"("State(s) in (\"\")"=w228) -> ("States Out"=w227:string)  [unwired: 14 in]
          }
          frame "Data: UI to UIconfig" {
            n86 = local read "Device Date"() -> (w245:string)
            n87 = local read "Username"() -> (w241:string)
            n88 = local read "Number of AI"() -> (w243:i32)
            n89 = local read "Lockin Address"() -> (w240:string)
            n90 = local read "KH Addresses"() -> (w238:refnum<visa-resource-name>[])
            n91 = local read "Strain Cell Address"() -> (w236:refnum<visa-resource-name>)
            n92 = local read "Capacitance Bridge Address"() -> (w234:refnum<visa-resource-name>)
            n93 = local read "Default Shunt Resistor"() -> (w233:T8)
            n94 = local read "Coupling"() -> (w249:T12)
            n95 = local read "Bandwidth Filter"() -> (w248:T11)
            n96 = local read "UI Channels []"() -> (w242:T1[])
            n97 = local read "Default Path"() -> (w247:path)
            n98 = local read "Default Gain"() -> (w231:T7)
            n99 = local read "Krohn Hite?"() -> (w239:bool)
            n100 = local read "Description"() -> (w244:string)
            n101 = local read "Strain Cell?"() -> (w237:bool)
            n102 = local read "Instrument"() -> (w232:T13)
            n103 = local read "C Bridge?"() -> (w235:bool)
            n104 = local read "Sample"() -> (w246:string)
            n105 = Bundle By Name(cluster=w230, "UIconfig.Metadata.Sample (SAXXXX)"=w246, "UIconfig.Metadata.Device (YYYYMMDD)"=w245, "UIconfig.Metadata.Description"=w244, "UIconfig.Metadata.Username"=w241, "UIconfig.Metadata.Default Path"=w247, "UIconfig.Number of AI"=w243, "UIconfig.UI Channels []"=w242, "UIconfig.Instruments.Lockin Address"=w240, "UIconfig.Instruments.Krohn Hite?"=w239, "UIconfig.Instruments.KH Addresses"=w238, "UIconfig.Instruments.Strain Cell?"=w237, "UIconfig.Instruments.Strain Cell Address"=w236, "UIconfig.Instruments.C Bridge?"=w235, "UIconfig.Instruments.Capacitance Bridge Address"=w234, "UIconfig.Instruments.Instrument"=w232, "UIconfig.Krohn Hite.Defualt Shunt Resistor"=w233, "UIconfig.Krohn Hite.Default Gain"=w231, "UIconfig.Krohn Hite.Coupling"=w249, "UIconfig.Krohn Hite.Bandwidth Filter"=w248) -> (w229:T19)
            n106 = call <vilib>:"Add State(s) to Queue__jki_lib_state_machine.vi"("State(s) in (\"\")"=w253) -> ("States Out"=w252:string)  [unwired: 14 in]
          }
          frame "Data: Cleanup" {
            # "Cleanup any data and references, here.\n(this is called automatically, by the Macro: Exit)"
            n107 = Unbundle By Name(w255) -> ("Core.Current VI Reference"=w258:refnum<vi>)
            n108 = Close Reference(reference=w258, error in (no error)=w257) -> (error out=w256:errorcluster)
            n109 = call <vilib>:"Add State(s) to Queue__jki_lib_state_machine.vi"("State(s) in (\"\")"=w260) -> ("States Out"=w259:string)  [unwired: 14 in]
          }
          frame "---------- UI ----------" {
            # "Do not put any code in this frame.\n(It is a separator no-op. You can make a copy of this frame to create a new UI frame)"
            n110 = call <vilib>:"Add State(s) to Queue__jki_lib_state_machine.vi"("State(s) in (\"\")"=w265) -> ("States Out"=w264:string)  [unwired: 14 in]
          }
          frame "UI: Initialize" {
            # "size window to decoration box on front panel"
            # "Initialize the User Interface, here.\n(this is called automatically, by the Macro: Init)"
            n111 = local write "Electrode Labels"("n.c\nI1+\nI1-\nI2+\nI2-\nI3+\nI3-\nV1+\nV1-\nV2+\nV2-\nV3+\nV3-\ndV1\ndV2\ndV3\nVsg1\nVsg2\nVsg3\nVsg4\nVbg" ("Electrode Labels")) -> ()
            n112 = call <userlib>:"Fit VI window to Largest Dec__ogtk.vi"("error in (no error)"=w270, "border spacing (2 px)"=0) -> ("error out"=w269:errorcluster)  [unwired: 4 in, 1 out]
            n113 = local write "Tab Control"(enum32{"Input", "Configuration", "UI", "Output"}."Input" ("Tab Control")) -> ()
            n114 = invoke on="STOP" class="Bool (strict)" method="Reinit To Default"() -> ()  [unwired: 3 in, 3 out]
            n115 = call <vilib>:"Add State(s) to Queue__jki_lib_state_machine.vi"("State(s) in (\"\")"=w274) -> ("States Out"=w273:string)  [unwired: 14 in]
          }
          frame "UI: Update Electrode Label Ring" {
            # "Update Electrode Label Ring"
            n116 = local read "Electrode Labels"() -> (w279:string)
            n117 = call <userlib>:"Multi-line String to Array__ogtk.vi"("string"=w279) -> ("lines"=w277:string[])
            n118 = control-ref of="Label"() -> (w278:refnum<vi>)
            n119 = property on="Property Node" class="Ring (strict)"(reference=w278, error in=w276, "Strings []"=w277) -> (error out=w275:errorcluster)  [unwired: 1 out]
            n120 = call <vilib>:"Add State(s) to Queue__jki_lib_state_machine.vi"("State(s) in (\"\")"=w283) -> ("States Out"=w282:string)  [unwired: 14 in]
          }
          frame "UI: Update KH Channel Ring" {
            # "Update KH Channel Ring"
            n121 = Unbundle By Name(w285) -> ("UIconfig.Number of AI"=w284:i32)
            n122 = call "Num AI Ch to KH Ch Labels.vi"("error in (no error)"=w289, "Number of AI"=w284) -> ("error out"=w290:errorcluster, "KH Ch []"=w286:string[])  [unwired: 8 in]
            n123 = control-ref of="Channel"() -> (w288:refnum<vi>)
            n124 = property on="Property Node" class="Ring (strict)"(reference=w288, error in=w290, "Strings []"=w286) -> (error out=w287:errorcluster)  [unwired: 1 out]
            n125 = call <vilib>:"Add State(s) to Queue__jki_lib_state_machine.vi"("State(s) in (\"\")"=w293) -> ("States Out"=w292:string)  [unwired: 14 in]
          }
          frame "UI: Initialize Channel Number" {
            # "Initialize Channel Number"
            n126 = Unbundle By Name(w299) -> ("UIconfig.Number of AI"=w294:i32, "UIconfig.UI Channels []"=w300:T1[])
            n127 = for {
              N: w294 -> [_]
              tunnel: w300 -> [w313]
              tunnel: [w310] -> w297 mode=indexing
              tunnel: "Default Shunt Resistor" -> [w307]
              tunnel: "Default Gain" -> [w306]
              i -> [w309]
              w311 = 1.0 ("AI.Gain")
              n128 = Increment(x=w309) -> (x+1=w308:i32)
              n129 = Index Array(array=w313, index=w309) -> (element=w312:T1)
              n130 = Bundle By Name(cluster=w312, "AI.Channel"=w308, "AI.Gain"=w311, "AO.Channel"=w308, "AO.Gain"=w311, "KH.Channel"=w308, "KH.Configuration"=Input_Configuration-Enum."Differential", "KH.Gain"=w306, "KH.Shunt Resistor"=w307) -> (w310:T1)
            }
            n131 = Bundle By Name(cluster=w299, "UI Channels []"=w297) -> (w298:T19)
            n132 = call <vilib>:"Add State(s) to Queue__jki_lib_state_machine.vi"("State(s) in (\"\")"=w304) -> ("States Out"=w303:string)  [unwired: 14 in]
          }
          frame "UI: Device Label to Configuration" {
            # "Convert Device Label (I,V,...) to KH Configuration (Differential, SE,...)"
            n133 = control-ref of="Label"() -> (w317:refnum<vi>)
            n134 = Unbundle By Name(w322) -> ("UI Channels []"=w320:T1[])
            n135 = property on="Property Node" class="Ring (strict)"(reference=w317, error in=w315) -> (error out=w316:errorcluster, "Strings []"=w318:string[])  [unwired: 1 out]
            n136 = for {
              tunnel: w320 -> [w330] mode=indexing
              tunnel: [w329] -> w319 mode=indexing
              tunnel: w318 -> [w328]
              shift-right: [w326] -> w314
              shift-left: w316 -> [w327]
              n137 = call "Device Label to Configuration.vi"("error in (no error)"=w327, "Ring Labels"=w328, "UI in"=w330) -> ("error out"=w326:errorcluster, "UI out"=w329:T1)  [unwired: 7 in]
            }
            n138 = Bundle By Name(cluster=w322, "UI Channels []"=w319) -> (w321:T19)
            n139 = call <vilib>:"Add State(s) to Queue__jki_lib_state_machine.vi"("State(s) in (\"\")"=w325) -> ("States Out"=w324:string)  [unwired: 14 in]
          }
          frame "UI: Dedupe KH" {
            # "remove duplicates"
            n140 = call-poly <userlib>:"Remove Duplicates from 1D Array__ogtk.vi"("Input Array"="KH Addresses") -> ("Output Array"=w335:variant[])  [unwired: 1 out]
            n141 = Variant To Data(error in=w333, type="KH Addresses", Variant=w335) -> (data=w332:refnum<visa-resource-name>[], error out=w331:errorcluster)
            n142 = local write "KH Addresses"(w332) -> ()
            n143 = call <vilib>:"Add State(s) to Queue__jki_lib_state_machine.vi"("State(s) in (\"\")"=w339) -> ("States Out"=w338:string)  [unwired: 14 in]
          }
          frame "UI: SR Disable" {
            # "#todo\nmove to SMO\nbut have public event to broadcast\nresistor value"
            # "#todo\nget this value from SMO"
            n144 = Unbundle By Name(w341) -> ("SR"=w340:enum16{"500", "10M"})
            n145 = control-ref of="Shunt Resistor"() -> (w344:refnum<vi>)
            n146 = call <userlib>:"Shunt - 500 or 10M Control Disable.vi"("error in"=w342, "SR"=w340, "reference"=w344) -> ("error out"=w346:errorcluster)  [unwired: 8 in]
            n147 = control-ref of="Defualt Shunt Resistor"() -> (w343:refnum<vi>)
            n148 = call <userlib>:"Shunt - 500 or 10M Control Disable.vi"("error in"=w346, "SR"=w340, "reference"=w343) -> ("error out"=w345:errorcluster)  [unwired: 8 in]
            n149 = call <vilib>:"Add State(s) to Queue__jki_lib_state_machine.vi"("State(s) in (\"\")"=w349) -> ("States Out"=w348:string)  [unwired: 14 in]
          }
          frame "UI: Blinking" {
            n150 = Equal?(x=w350, y="True") -> (x = y?=w351:bool)
            n151 = control-ref of="Blinking String"() -> (w353:refnum<vi>)
            n152 = property on="Property Node" class="Str"(reference=w353, "Blinking"=w351) -> ()  [unwired: 1 in, 2 out]
            n153 = call <vilib>:"Add State(s) to Queue__jki_lib_state_machine.vi"("State(s) in (\"\")"=w358) -> ("States Out"=w357:string)  [unwired: 14 in]
          }
          frame "UI: Show Hide Instruments" {
            n154 = control-ref of="KH Addresses"() -> (w366:refnum<vi>)
            n155 = control-ref of="Capacitance Bridge Address"() -> (w365:refnum<vi>)
            n156 = control-ref of="Strain Cell Address"() -> (w364:refnum<vi>)
            n157 = Build Array(w366, w365, w364) -> (w360:refnum<vi>[])
            n158 = Build Array("Krohn Hite?", "C Bridge?", "Strain Cell?") -> (w359:bool[])
            n159 = for {
              tunnel: w360 -> [w373] mode=indexing
              tunnel: w359 -> [w372] mode=indexing
              n160 = property on="Property Node" class="Ctl"(reference=w373, "Visible"=w372) -> ()  [unwired: 1 in, 2 out]
            }
            n161 = call <vilib>:"Add State(s) to Queue__jki_lib_state_machine.vi"("State(s) in (\"\")"=w371) -> ("States Out"=w370:string)  [unwired: 14 in]
          }
          frame "UI: UIconfig to UI" {
            n162 = Unbundle By Name(w393) -> ("UIconfig.Metadata.Sample (SAXXXX)"=w389:string, "UIconfig.Metadata.Device (YYYYMMDD)"=w388:string, "UIconfig.Metadata.Description"=w387:string, "UIconfig.Metadata.Username"=w384:string, "UIconfig.Metadata.Default Path"=w390:path, "UIconfig.Number of AI"=w386:i32, "UIconfig.UI Channels []"=w385:T1[], "UIconfig.Instruments.Lockin Address"=w383:string, "UIconfig.Instruments.Krohn Hite?"=w382:bool, "UIconfig.Instruments.KH Addresses"=w381:refnum<visa-resource-name>[], "UIconfig.Instruments.Strain Cell?"=w380:bool, "UIconfig.Instruments.Strain Cell Address"=w379:refnum<visa-resource-name>, "UIconfig.Instruments.C Bridge?"=w378:bool, "UIconfig.Instruments.Capacitance Bridge Address"=w377:refnum<visa-resource-name>, "UIconfig.Instruments.Instrument"=w375:T13, "UIconfig.Krohn Hite.Defualt Shunt Resistor"=w376:T8, "UIconfig.Krohn Hite.Default Gain"=w374:T7, "UIconfig.Krohn Hite.Coupling"=w392:T12, "UIconfig.Krohn Hite.Bandwidth Filter"=w391:T11)
            n163 = local write "Sample"(w389) -> ()
            n164 = local write "Description"(w387) -> ()
            n165 = local write "Default Path"(w390) -> ()
            n166 = local write "UI Channels []"(w385) -> ()
            n167 = local write "Krohn Hite?"(w382) -> ()
            n168 = local write "Strain Cell?"(w380) -> ()
            n169 = local write "C Bridge?"(w378) -> ()
            n170 = local write "Instrument"(w375) -> ()
            n171 = local write "Default Gain"(w374) -> ()
            n172 = local write "Bandwidth Filter"(w391) -> ()
            n173 = local write "Capacitance Bridge Address"(w377) -> ()
            n174 = local write "Default Shunt Resistor"(w376) -> ()
            n175 = local write "Strain Cell Address"(w379) -> ()
            n176 = local write "Lockin Address"(w383) -> ()
            n177 = local write "Number of AI"(w386) -> ()
            n178 = local write "KH Addresses"(w381) -> ()
            n179 = local write "Device Date"(w388) -> ()
            n180 = local write "Username"(w384) -> ()
            n181 = local write "Coupling"(w392) -> ()
            n182 = call <vilib>:"Add State(s) to Queue__jki_lib_state_machine.vi"("State(s) in (\"\")"=w397) -> ("States Out"=w396:string)  [unwired: 14 in]
          }
          frame "UI: Update UI Array" {
            n183 = Unbundle By Name(w399) -> ("UI Channels []"=w398:T1[])
            n184 = local write "UI Channels []"(w398) -> ()
            n185 = call <vilib>:"Add State(s) to Queue__jki_lib_state_machine.vi"("State(s) in (\"\")"=w403) -> ("States Out"=w402:string)  [unwired: 14 in]
          }
          frame "UI: Cursor Set" {
            # "Argument"
            # "Initialize the User Interface, here.\n(this is called automatically, by the Macro: Init)"
            n186 = disable-structure shown="Default" {
              disable-tunnel: w406 -> [w411 w414]
              disable-tunnel: [w411 w413] -> w405
              disable-tunnel: w404 -> [_ w412]
              frame condition #0 {
              }
              frame condition #1 (active) {
                n187 = case shown="\"Busy\"" w412 {
                  tunnel: w414 -> [w416 w418]
                  tunnel: [w415 w417] -> w413
                  frame "Idle", Default {
                    n188 = call <vilib>:"Unset Busy.vi"("error in (no error)"=w416) -> ("error out"=w415:errorcluster)  [unwired: 10 in]
                  }
                  frame "Busy" {
                    n189 = call <vilib>:"Set Busy.vi"("error in (no error)"=w418) -> ("error out"=w417:errorcluster)  [unwired: 9 in, 1 out]
                  }
                }
              }
            }
            n190 = call <vilib>:"Add State(s) to Queue__jki_lib_state_machine.vi"("State(s) in (\"\")"=w410) -> ("States Out"=w409:string)  [unwired: 14 in]
          }
          frame "UI: Front Panel State" {
            # "Argument"
            # "Set Front Panel Open or Closed\n(Usage: \"UI: Front Panel State >> Open|Close\")"
            n191 = Unbundle By Name(w422) -> ("Core.Current VI Reference"=w421:refnum<vi>)
            n192 = disable-structure shown="Default" {
              disable-tunnel: w424 -> [w430 w453]
              disable-tunnel: [w429 w453] -> w423
              disable-tunnel: w421 -> [w428 _]
              disable-tunnel: w420 -> [w427 _]
              frame condition #0 (active) {
                n193 = case shown="\"Close\"" w427 {
                  tunnel: w430 -> [w434 w447]
                  tunnel: [w436 w448] -> w429
                  tunnel: w428 -> [w435 w445]
                  frame "Open", Default {
                    n194 = property class="VI"(reference=w435, error in=w434) -> (reference out=w432:refnum<vi>, error out=w433:errorcluster, "FP.State"=w431:T16)
                    n195 = case shown="\"Closed\"" w431 {
                      tunnel: [w439 w442] -> w436
                      tunnel: w433 -> [w438 w442]
                      tunnel: w432 -> [w437 _]
                      frame "Closed" {
                        n196 = invoke class="VI" method="FP.Open"(reference=w437, error in=w438, "Activate"=TRUE, "State"=T16."Standard") -> (error out=w439:errorcluster)  [unwired: 1 in, 4 out]
                      }
                      frame Default {
                      }
                    }
                  }
                  frame "Close" {
                    n197 = property class="VI"(reference=w445, error in=w447) -> (reference out=w444:refnum<vi>, error out=w446:errorcluster, "FP.State"=w443:T16)
                    n198 = case shown="Default" w443 {
                      tunnel: [w449 w452] -> w448
                      tunnel: w446 -> [w449 w451]
                      tunnel: w444 -> [_ w450]
                      frame "Invalid", "Closed" {
                      }
                      frame Default {
                        n199 = invoke class="VI" method="FP.Close"(reference=w450, error in=w451) -> (error out=w452:errorcluster)  [unwired: 1 in, 2 out]
                      }
                    }
                  }
                }
              }
              frame condition #1 {
              }
            }
            n200 = call <vilib>:"Add State(s) to Queue__jki_lib_state_machine.vi"("State(s) in (\"\")"=w426) -> ("States Out"=w425:string)  [unwired: 14 in]
          }
          frame "---------- Macro ----------" {
            n201 = call <vilib>:"Add State(s) to Queue__jki_lib_state_machine.vi"("State(s) in (\"\")"=w458) -> ("States Out"=w457:string)  [unwired: 14 in]
          }
          frame "Macro: Initialize" {
            # "Initialization Macro\n(This is called once, when the VI starts)"
            n202 = call <vilib>:"Add State(s) to Queue__jki_lib_state_machine.vi"("State(s) in Front (\"\")"="Data: Initialize\nInitialize Core Data\nEvents: Register", "State(s) in (\"\")"="Process: Sync", "State(s) at Back (\"\")"="UI: Initialize\nUI: Front Panel State >> Open\nMacro: Initialize UI") -> ("States Out"=w460:string)  [unwired: 12 in]
            n203 = call <vilib>:"Add State(s) to Queue__jki_lib_state_machine.vi"("State(s) in Front (\"\")"=w460, "State(s) in (\"\")"=w467) -> ("States Out"=w466:string)  [unwired: 13 in]
          }
          frame "Macro: Initialize UI" {
            n204 = call <vilib>:"Add State(s) to Queue__jki_lib_state_machine.vi"("State(s) in Front (\"\")"="UI: Update Electrode Label Ring\nUI: Update KH Channel Ring\nUI: Initialize Channel Number\nUI: Device Label to Configuration\nUI: Update UI Array\nUI: Show Hide Instruments\nExperiment VIs: Populate VI Ring" ("State(s) in Front (\"\")"), "State(s) in (\"\")"=w473) -> ("States Out"=w472:string)  [unwired: 13 in]
          }
          frame "Macro: Output" {
            n205 = call <vilib>:"Add State(s) to Queue__jki_lib_state_machine.vi"("State(s) in Front (\"\")"="Data: UI to UIconfig\nAction: setUIconfig" ("State(s) in Front (\"\")"), "State(s) in (\"\")"=w479) -> ("States Out"=w478:string)  [unwired: 13 in]
          }
          frame "Macro: Exit" {
            # "Exit Macro\n(This is called once, when the VI exits)"
            n206 = Unbundle By Name(w481) -> ("Core.Close Panel on Exit?"=w491:bool)
            n207 = Select(t="UI: Front Panel State >> Close", s=w491, f="") -> (s? t:f=w488:string)
            n208 = call <vilib>:"Add State(s) to Queue__jki_lib_state_machine.vi"("State(s) in Front (\"\")"="Data: Cleanup\nEvents: Unregister\nProcess: Self Terminate", "State(s) in (\"\")"="Process: Sync", "State(s) at Back (\"\")"="Exit") -> ("States Out"=w483:string)  [unwired: 12 in]
            n209 = call <vilib>:"Add State(s) to Queue__jki_lib_state_machine.vi"("State(s) in Front (\"\")"="", "State(s) in (\"\")"=w488, "State(s) at Back (\"\")"=w483) -> ("States Out"=w487:string)  [unwired: 12 in]
            n210 = call <vilib>:"Add State(s) to Queue__jki_lib_state_machine.vi"("State(s) in Front (\"\")"=w487, "State(s) in (\"\")"=w494) -> ("States Out"=w493:string)  [unwired: 13 in]
          }
          frame "---------- Process ----------" {
            # "Template Separator\n(You can make a copy of, or modify, this frame)"
            n211 = call <vilib>:"Add State(s) to Queue__jki_lib_state_machine.vi"("State(s) in (\"\")"=w499) -> ("States Out"=w498:string)  [unwired: 14 in]
          }
          frame "Process: Sync" {
            n212 = Unbundle By Name(w507) -> ("Instrument UI"=w503:refnum<class "Control Experiment UI.lvclass">)
            n213 = call <vilib>:"WaitOnProcessSync.vi"("error in (no error)"=w502, "SMO"=w503) -> ("error out"=w501:errorcluster, "Don't run?"=w506:bool)  [unwired: 7 in, 1 out]
            n214 = Select(t="Data: Cleanup\nEvents: Unregister\nExit", s=w506, f="") -> (s? t:f=w500:string)
            n215 = call <vilib>:"Add State(s) to Queue__jki_lib_state_machine.vi"("State(s) in Front (\"\")"=w500, "State(s) in (\"\")"=w510) -> ("States Out"=w509:string)  [unwired: 13 in]
          }
          frame "Process: Self Terminate" {
            n216 = Unbundle By Name(w512) -> ("Instrument UI"=w511:refnum<class "Control Experiment UI.lvclass">)
            n217 = call <vilib>:"SelfTerminate.vi"("error in (no error)"=w514, "SMO in"=w511) -> ("error out"=w513:errorcluster)  [unwired: 8 in, 1 out]
            n218 = call <vilib>:"Add State(s) to Queue__jki_lib_state_machine.vi"("State(s) in (\"\")"=w517) -> ("States Out"=w516:string)  [unwired: 14 in]
          }
          frame "---------- Events ----------" {
            # "Template Separator\n(You can make a copy of, or modify, this frame)"
            n219 = call <vilib>:"Add State(s) to Queue__jki_lib_state_machine.vi"("State(s) in (\"\")"=w522) -> ("States Out"=w521:string)  [unwired: 14 in]
          }
          frame "Events: Register" {
            # "Expand to add\nmore events"
            # "Base Class Protected Events"
            n220 = Unbundle By Name(w536) -> ("Instrument UI"=w526:refnum<class "Control Experiment UI.lvclass">, "Instrument"=w529:refnum<class "Control Experiment.lvclass">)
            n221 = call <vilib>:"GetProtectedEvents.vi"("SMO"=w526) -> ("error out"=w530:errorcluster, "SMO Protected Events"=w534:T22)  [unwired: 8 in, 1 out]
            n222 = call <userlib>:"Instrument.GetPublicEvents.vi"("Instrument"=w529) -> ("error out"=w527:errorcluster, "Instrument Public Events"=w528:T23, "Instrument out"=w525:refnum<class "Control Experiment.lvclass">)  [unwired: 8 in]
            n223 = call "Control Experiment.GetPublicEvents.vi"("Control Experiment"=w525) -> ("error out"=w523:errorcluster, "Public Events"=w524:T24)  [unwired: 8 in, 1 out]
            n224 = register-events(w534, w528, w524) -> (reference out=w535:refnum<event-registration>, error out=w532:errorcluster)  [unwired: 2 in]
            n225 = Merge Errors(w523, w527, w533, w532, w530) -> (w531:errorcluster)
            n226 = call <vilib>:"Add State(s) to Queue__jki_lib_state_machine.vi"("State(s) in (\"\")"=w538) -> ("States Out"=w537:string)  [unwired: 14 in]
          }
          frame "Events: Unregister" {
            n227 = Unregister For Events(event registration refnum=w541, error in=w540) -> (error out=w539:errorcluster)
            n228 = call <vilib>:"Add State(s) to Queue__jki_lib_state_machine.vi"("State(s) in (\"\")"=w544) -> ("States Out"=w543:string)  [unwired: 14 in]
          }
          frame "---------- Action ----------" {
            n229 = Unbundle By Name(w547) -> ("Instrument UI"=w545:refnum<class "Control Experiment UI.lvclass">)
            n230 = Bundle By Name(cluster=w547, "Instrument UI"=w545) -> (w546:T19)
            n231 = call <vilib>:"Add State(s) to Queue__jki_lib_state_machine.vi"("State(s) in (\"\")"=w551) -> ("States Out"=w550:string)  [unwired: 14 in]
          }
          frame "Action: Notify UI Closed" {
            # "Notify that the UI has been closed"
            n232 = Unbundle By Name(w554) -> ("Instrument UI"=w555:refnum<class "Control Experiment UI.lvclass">)
            n233 = call <vilib>:"Hide.vi"("error in (no error)"=w553, "SMO.UI"=w555) -> ("error out"=w552:errorcluster)  [unwired: 8 in, 1 out]
            n234 = call <vilib>:"Add State(s) to Queue__jki_lib_state_machine.vi"("State(s) in (\"\")"=w558) -> ("States Out"=w557:string)  [unwired: 14 in]
          }
          frame "Action: setUIconfig" {
            n235 = Unbundle By Name(w563) -> ("Instrument"=w562:refnum<class "Control Experiment.lvclass">, "UIconfig"=w561:T17)
            n236 = call "Control Experiment.setUIconfig.vi"("error in (no error)"=w560, "UI Configuration"=w561, "Control Experiment"=w562) -> ("error out"=w559:errorcluster)  [unwired: 7 in, 1 out]
            n237 = call <vilib>:"Add State(s) to Queue__jki_lib_state_machine.vi"("State(s) in (\"\")"=w566) -> ("States Out"=w565:string)  [unwired: 14 in]
          }
          frame "Action: saveKHpreset" {
            n238 = Unbundle By Name(w571) -> ("Instrument"=w570:refnum<class "Control Experiment.lvclass">)
            n239 = call "Control Experiment.saveKHpreset.vi"("error in (no error)"=w569, "saveKHpreset"=w567, "Control Experiment"=w570) -> ("error out"=w568:errorcluster)  [unwired: 7 in, 1 out]
            n240 = call <vilib>:"Add State(s) to Queue__jki_lib_state_machine.vi"("State(s) in (\"\")"=w574) -> ("States Out"=w573:string)  [unwired: 14 in]
          }
          frame "Action: loadKHpreset" {
            n241 = Unbundle By Name(w579) -> ("Instrument"=w578:refnum<class "Control Experiment.lvclass">)
            n242 = call "Control Experiment.loadKHpreset.vi"("error in (no error)"=w577, "loadKHpreset"=w575, "Control Experiment"=w578) -> ("error out"=w576:errorcluster)  [unwired: 7 in, 1 out]
            n243 = call <vilib>:"Add State(s) to Queue__jki_lib_state_machine.vi"("State(s) in (\"\")"=w582) -> ("States Out"=w581:string)  [unwired: 14 in]
          }
          frame "---------- Experiment VIs ----------" {
            n244 = Unbundle By Name(w585) -> ("Instrument UI"=w584:refnum<class "Control Experiment UI.lvclass">)
            n245 = Bundle By Name(cluster=w585, "Instrument UI"=w584) -> (w583:T19)
            n246 = call <vilib>:"Add State(s) to Queue__jki_lib_state_machine.vi"("State(s) in (\"\")"=w589) -> ("States Out"=w588:string)  [unwired: 14 in]
          }
          frame "Experiment VIs: Populate VI Ring" {
            # "Populate the Ring with a list of Experiment VIs"
            n247 = call <userlib>:"Current VIs Parent Directory__ogtk.vi"() -> ("Parent Directory (+ Relative)"=w605:path)  [unwired: 5 in]
            n248 = call <userlib>:"String to 1D Array__ogtk.vi"("delimiter (Tab)"="\n", "string"="----Sweep Control----\nSweep Control.vi\nContinuous B Sweep.vi") -> ("Array of Strings"=w594:string[])  [unwired: 9 in]
            n249 = call <userlib>:"String to 1D Array__ogtk.vi"("delimiter (Tab)"="\n", "string"="----Transport----\nIV.vi\nIV_Sweep.vi\nLockin_time.vi\nLockin_Vsg.vi\nLockin_sweep.vi\nLockin_AIWFM_time.vi\nTHz_TimeDelay.vi\nSweep_AIWFM_time.vi") -> ("Array of Strings"=w593:string[])  [unwired: 9 in]
            n250 = Strip Path(path=w605) -> (stripped path=w602:path)  [unwired: 1 out]
            n251 = Build Path(base path=w602, name or relative path="SweepControl") -> (appended path=w601:path)
            n252 = Build Path(base path=w602, name or relative path="Transport") -> (appended path=w597:path)
            n253 = for {
              tunnel: w601 -> [w618]
              tunnel: w594 -> [w617] mode=indexing
              tunnel: [w616] -> w596 mode=indexing
              n254 = Build Path(base path=w618, name or relative path=w617) -> (appended path=w616:path)
            }
            n255 = for {
              tunnel: w597 -> [w615]
              tunnel: w593 -> [w614] mode=indexing
              tunnel: [w613] -> w595 mode=indexing
              n256 = Build Path(base path=w615, name or relative path=w614) -> (appended path=w613:path)
            }
            n257 = control-ref of="Experiment VIs"() -> (w590:refnum<vi>)
            n258 = Build Array (concatenate)(w596, w595) -> (w592:path[])
            n259 = Build Array (concatenate)(w594, w593) -> (w591:string[])
            n260 = property on="Property Node" class="Ring (strict)"(reference=w590, "Strings []"=w591) -> ()  [unwired: 1 in, 2 out]
            n261 = Bundle By Name(cluster=w608, "VI paths"=w592) -> (w607:T19)
            n262 = call <vilib>:"Add State(s) to Queue__jki_lib_state_machine.vi"("State(s) in (\"\")"=w612) -> ("States Out"=w611:string)  [unwired: 14 in]
          }
          frame "Experiment VIs: Open VI" {
            # "Opens Transport VIs on this machine"
            n263 = Unbundle By Name(w619) -> ("VI paths"=w624:path[])
            n264 = Index Array(array=w624, index="Experiment VIs") -> (element=w622:path)
            n265 = call "Open Experiment VI.vi"("error in (no error)"=w621, "Path"=w622) -> ("error out"=w620:errorcluster)  [unwired: 9 in]
            n266 = call <vilib>:"Add State(s) to Queue__jki_lib_state_machine.vi"("State(s) in (\"\")"=w627) -> ("States Out"=w626:string)  [unwired: 14 in]
          }
          frame "Experiment VIs: Open Lockin" {
            # "Opens the Lockin Application on this machine"
            n267 = call "Open Lockin.vi"("error in (no error)"=w629) -> ("error out"=w628:errorcluster)  [unwired: 10 in]
            n268 = call <vilib>:"Add State(s) to Queue__jki_lib_state_machine.vi"("State(s) in (\"\")"=w633) -> ("States Out"=w632:string)  [unwired: 14 in]
          }
          frame "---------- KH ----------" {
            n269 = Unbundle By Name(w636) -> ("Instrument UI"=w635:refnum<class "Control Experiment UI.lvclass">)
            n270 = Bundle By Name(cluster=w636, "Instrument UI"=w635) -> (w634:T19)
            n271 = call <vilib>:"Add State(s) to Queue__jki_lib_state_machine.vi"("State(s) in (\"\")"=w640) -> ("States Out"=w639:string)  [unwired: 14 in]
          }
          frame "KH: Set Channels" {
            # "keep here...\n#todo\nneed method to send UI channels to SMO\nand KH channels to SMO\n(or move this method to SMO?)"
            n272 = Unbundle By Name(w644) -> ("UI Channels []"=w645:T1[])
            n273 = local read "Default Shunt Resistor"() -> (w647:T8)
            n274 = call "UI Array act All Buttons.vi"("error in (no error)"=w646, "Default Shunt Resistor"=w647, "KH All Buttons"="KH All Buttons", "UI Channels []"=w645) -> ("error out"=w641:errorcluster, "UI Channels [] out"=w642:T1[])  [unwired: 6 in]
            n275 = flat-sequence {
              tunnel: w641 -> [_]
              frame #0 {
                n276 = local write "KH All Buttons"(T10."No Selection" ("KH All Buttons")) -> ()
              }
            }
            n277 = Bundle By Name(cluster=w644, "UI Channels []"=w642) -> (w643:T19)
            n278 = call <vilib>:"Add State(s) to Queue__jki_lib_state_machine.vi"("State(s) in (\"\")"=w651) -> ("States Out"=w650:string)  [unwired: 14 in]
          }
        }
      }
    }
    frame Error {
    }
  }
  n279 = call-parent "Process.vi"("error in"=w8, "Instrument UI in"=w7) -> ("error out"=w5:errorcluster, "Instrument UI out"=→"Sequence Experiment UI out":refnum<class "Control Experiment UI.lvclass">)  [unwired: 8 in]
  n280 = Merge Errors(w5, w4) -> (→"error out":errorcluster)
  n281 = disable-structure shown="Disabled" {
    frame Disabled {
      n282 = call "JSON DIDDLE.vi"() -> ()  [unwired: 12 in]
    }
    frame Enabled {
    }
  }
